vi "Power Factor Non Linear Load (SubVI).vi"(9 "apparent power [VA]":dbl, 10 "Dynamic Data":dynamicdata(waveform), 11 "Dynamic Data 2":dynamicdata(waveform)) -> (3 "Power Factor":dbl[](array[numeric]))   [LabVIEW 2015]
uses:
  <vilib>/measure/matone.llb/Extract Single Tone Information N Chan.vi
  <vilib>/measure/NI_MAPro.lvlib
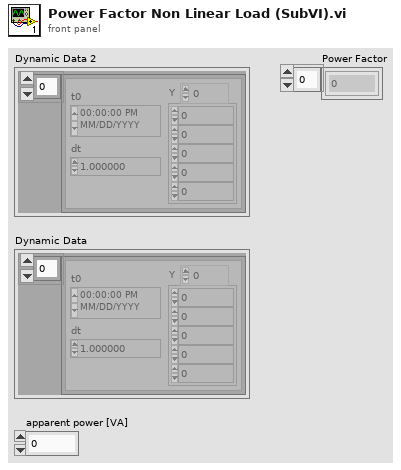
[diagram p1: front panel]
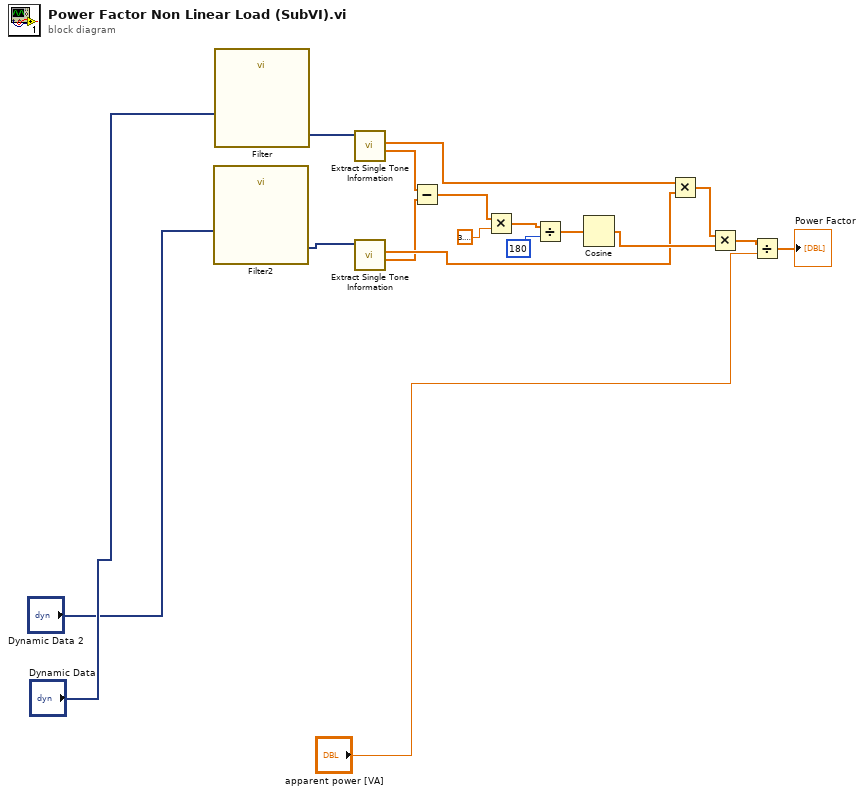
[diagram p0: block diagram]
diagram:
  n1 = call "Filter2"("Signal"="Dynamic Data 2") -> ("Filtered Signal"=w4:dynamicdata)  [unwired: 9 in, 1 out]
  n2 = call "Filter"("Signal"="Dynamic Data") -> ("Filtered Signal"=w3:dynamicdata)  [unwired: 9 in, 1 out]
  n3 = call-poly <vilib>:"Extract Single Tone Information.vi"("time signals in"=w3) -> ("detected phases (deg)"=w5:dbl[], "detected amplitudes"=w12:dbl[])  [unwired: 5 in, 4 out]
  n4 = call-poly <vilib>:"Extract Single Tone Information.vi"("time signals in"=w4) -> ("detected phases (deg)"=w6:dbl[], "detected amplitudes"=w13:dbl[])  [unwired: 5 in, 4 out]
  n5 = Subtract(x=w5, y=w6) -> (x-y=w7:dbl[])
  n6 = Multiply(x=w7, y=3.141592653589793) -> (x*y=w9:dbl[])
  n7 = Divide(x=w9, y=180) -> (x/y=w11:dbl[])
  n8 = Cosine(x=w11) -> (cos(x)=w15:dbl[])
  n9 = Multiply(x=w12, y=w13) -> (x*y=w14:dbl[])
  n10 = Multiply(x=w14, y=w15) -> (x*y=w16:dbl[])
  n11 = Divide(x=w16, y="apparent power [VA]") -> (x/y=→"Power Factor":dbl[])
